vi "sv_Calculate Chirp Time and Phase Relation within Block.vi"(6 "# of even-angle samples in":i32, 10 "block size [samples]":i32, 11 "continuous swept-sine settings":T1={"amplitude"=0.0, "frequency range"={"start (Hz)"=20.0, "stop (Hz)"=20000.0, "frequency spacing"=enum."Logarithmic"}, "sampling info"={"Fs"=50000.0, "chirp duration [s]"=3.0}, "initial states"={"frequency [Hz]"=20.0, "phase [rad]"=0.0, "elapsed time [s]"=0.0}, "frequency slope"=0.0, "maximum harmonic"=0, "prefix len [samples]"={"integer"=0, "fractional"=0.0}} {"frequency slope" format="%.2f"; "prefix len [samples]"."fractional" format="%.2p"; "initial states"."elapsed time [s]" format="%.2f"; "initial states"."phase [rad]" format="%.2f"; "initial states"."frequency [Hz]" format="%.2f"; "sampling info"."chirp duration [s]" format="%.2f"; "sampling info"."Fs" format="%.2p"; "frequency range"."stop (Hz)" format="%.2f"; "frequency range"."start (Hz)" format="%.2f"; "amplitude" format="%.2f"}) -> (0 "samples/rev":i32, 1 "time instances [s]":dbl[](array[numeric]), 2 "phases [rad]":dbl[](array[numeric]), 3 "continuous swept-sine settings out":T1={"amplitude"=0.0, "frequency range"={"start (Hz)"=20.0, "stop (Hz)"=20000.0, "frequency spacing"=enum."Logarithmic"}, "sampling info"={"Fs"=50000.0, "chirp duration [s]"=3.0}, "initial states"={"frequency [Hz]"=20.0, "phase [rad]"=0.0, "elapsed time [s]"=0.0}, "frequency slope"=0.0, "maximum harmonic"=0, "prefix len [samples]"={"integer"=0, "fractional"=0.0}} {"frequency slope" format="%.2f"; "prefix len [samples]"."fractional" format="%.2p"; "initial states"."elapsed time [s]" format="%.2f"; "initial states"."phase [rad]" format="%.2f"; "initial states"."frequency [Hz]" format="%.2f"; "sampling info"."chirp duration [s]" format="%.2f"; "sampling info"."Fs" format="%.2p"; "frequency range"."stop (Hz)" format="%.2f"; "frequency range"."start (Hz)" format="%.2f"; "amplitude" format="%.2f"}, 4 "# of even-angle samples out":i32)   [LabVIEW 2017, in "SoundVib_ContSweptSine.lvlib"]
uses:
  <vilib>/addons/Sound and Vibration/svt_Continuous Swept Sine/SoundVib_ContSweptSine.lvlib
  <vilib>/addons/_NISVFA/_Generation/subVIs/sv_Chirp Settings.ctl
  <vilib>/Analysis/1siggen.llb/Ramp Pattern by Samples.vi
  <vilib>/addons/_NISVFA/_Generation/SoundVib_Generation.lvlib
  <vilib>/Analysis/NI_AALBase.lvlib
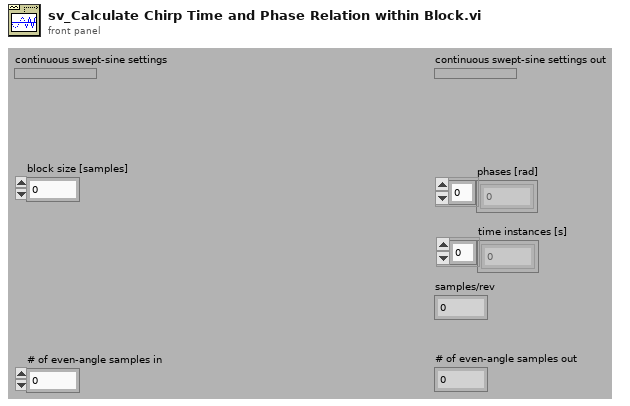
[diagram p1: front panel]
types:
  T1 = typedef "SoundVib_Generation.lvlib/sv_Chirp Settings.ctl" = cluster{"amplitude":dbl, "frequency range":cluster{"start (Hz)":dbl, "stop (Hz)":dbl, "frequency spacing":enum16{"Linear", "Logarithmic"}}, "sampling info":cluster{"Fs":dbl, "chirp duration [s]":dbl}, "initial states":cluster{"frequency [Hz]":dbl, "phase [rad]":dbl, "elapsed time [s]":dbl}, "frequency slope":dbl, "maximum harmonic":i32, "prefix len [samples]":cluster{"integer":u32, "fractional":dbl}}
  T2 = cluster{"frequency [Hz]":dbl, "phase [rad]":dbl, "elapsed time [s]":dbl}
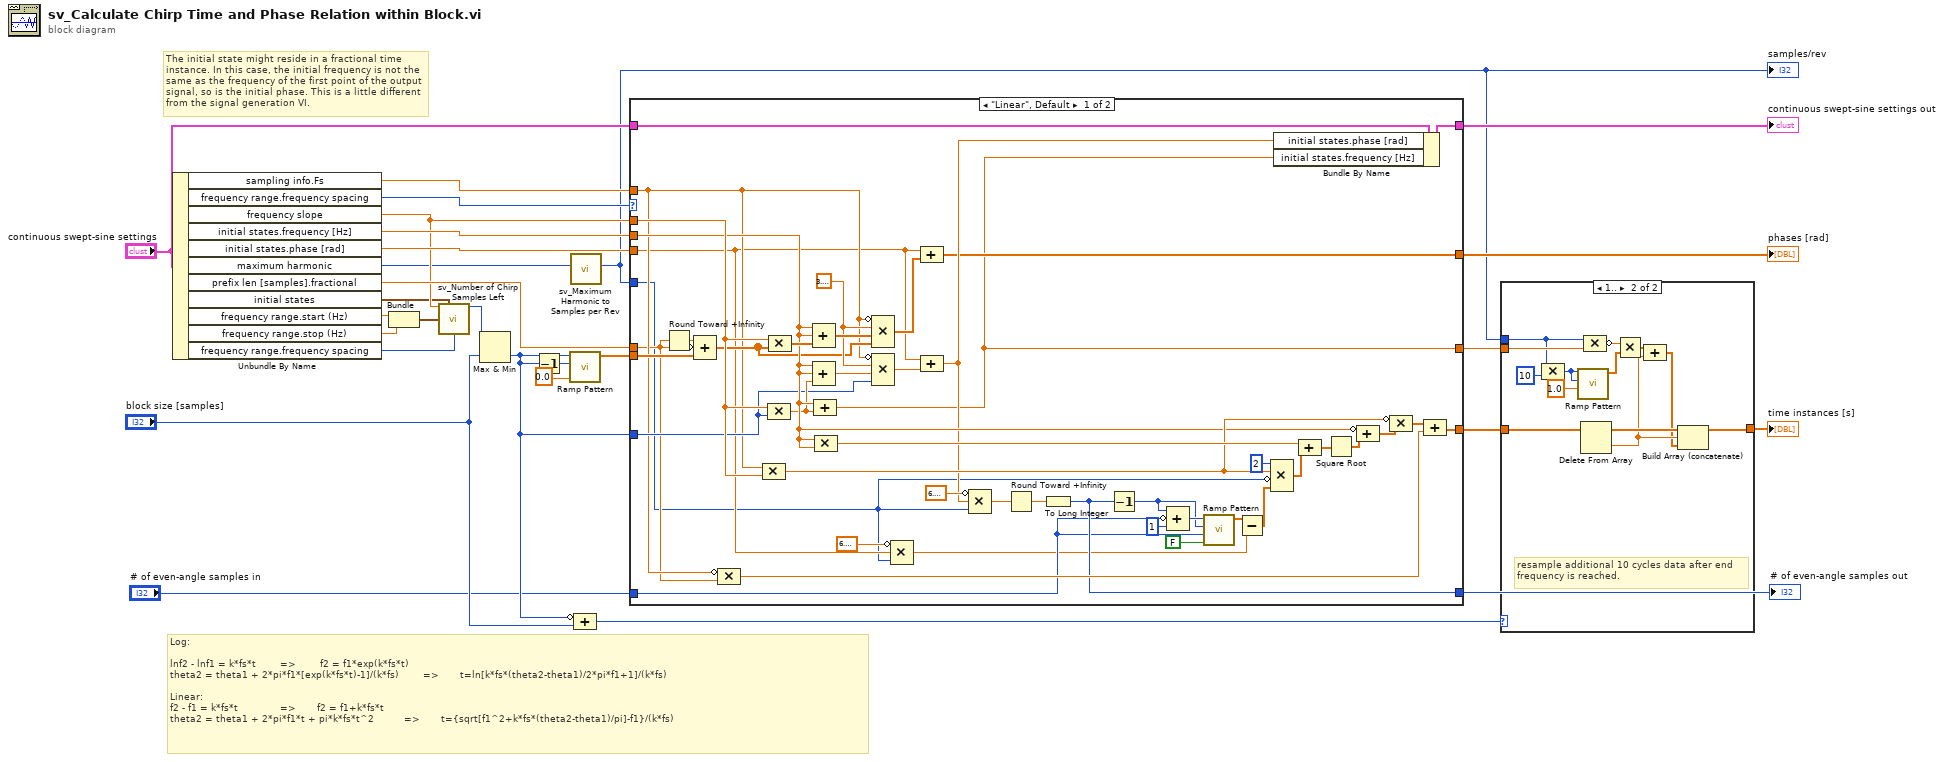
[diagram p0: block diagram]
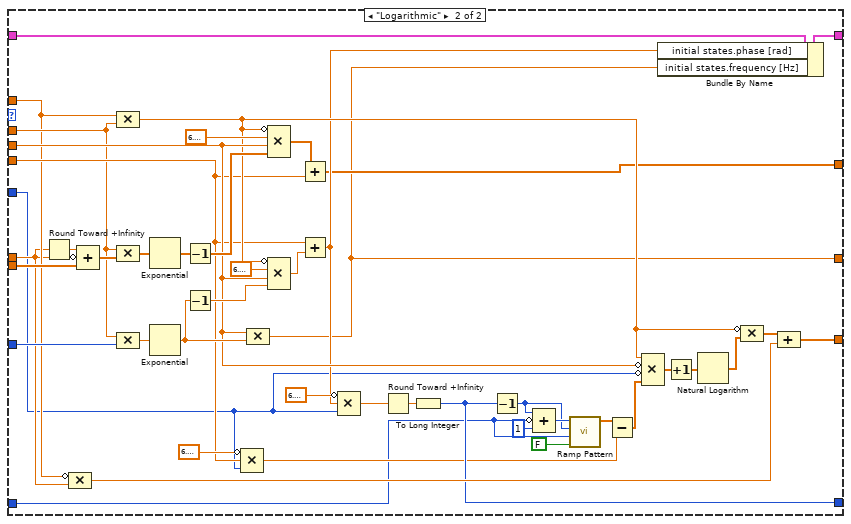
[diagram p3: hidden frame]
diagram:
  # "The initial state might reside in a fractional time instance. In this case, the initial frequency is not the same as the frequency of the first point of the output signal, so is the initial phase. This is a little different from the signal generation VI."
  # "Log:\n            \nlnf2 - lnf1 = k*fs*t        =>        f2 = f1*exp(k*fs*t)\ntheta2 = theta1 + 2*pi*f1*[exp(k*fs*t)-1]/(k*fs)        =>       t=ln[k*fs*(theta2-theta1)/2*pi*f1+1]/(k*fs)\n\nLinear:\nf2 - f1 = k*fs*t              =>       f2 = f1+k*fs*t\ntheta2 = theta1 + 2*pi*f1*t + pi*k*fs*t^2          =>       t={sqrt[f1^2+k*fs*(theta2-theta1)/pi]-f1}/(k*fs)"
  n1 = Unbundle By Name("continuous swept-sine settings") -> ("sampling info.Fs"=w16:dbl, "frequency range.frequency spacing"=w28:enum16{"Linear", "Logarithmic"}, "frequency slope"=w19:dbl, "initial states.frequency [Hz]"=w27:dbl, "initial states.phase [rad]"=w26:dbl, "maximum harmonic"=w4:i32, "prefix len [samples].fractional"=w21:dbl, "initial states"=w18:T2, "frequency range.start (Hz)"=w7:dbl, "frequency range.stop (Hz)"=w6:dbl, "frequency range.frequency spacing"=w5:enum16{"Linear", "Logarithmic"})
  n2 = Bundle("start (Hz)"=w7, "stop (Hz)"=w6) -> (w8:cluster{"start (Hz)":dbl, "stop (Hz)":dbl})  [unwired: 1 in]
  n3 = call <vilib>:"sv_Number of Chirp Samples Left.vi"("frequency slope"=w19, "initial states"=w18, "frequency range"=w8, "frequency spacing"=w5) -> ("# of samples left"=w17:i32)  [unwired: 9 in, 2 out]
  n4 = Max & Min(x=w17, y="block size [samples]") -> (min(x,y)=w14:i32)  [unwired: 1 out]
  n5 = Decrement(x=w14) -> (x-1=w20:i32)
  n6 = call-poly <vilib>:"Ramp Pattern.vi"("start"=0.0, "end"=w20, "samples"=w14) -> ("Ramp Pattern"=w24:dbl[])  [unwired: 7 in, 1 out]
  n7 = call <vilib>:"sv_Maximum Harmonic to Samples per Rev.vi"("maximum harmonic"=w4) -> ("samples/rev"=w3:i32)  [unwired: 10 in]
  "samples/rev" <- w3
  n8 = Compound Arithmetic op=ADD(invert w14, "block size [samples]") -> (w12:i32)
  n9 = case shown="\"Linear\", Default" w28 {
    tunnel: w27 -> [w53 w96]
    tunnel: w26 -> [w36 w93]
    tunnel: w19 -> [w62 w83]
    tunnel: w24 -> [w43 w115]
    tunnel: "continuous swept-sine settings" -> [w71 w116]
    tunnel: [w45 w90] -> w15
    tunnel: w14 -> [w47 w114]
    tunnel: [w70 w110] -> w22
    tunnel: w16 -> [w39 w82]
    tunnel: w3 -> [w30 w76]
    tunnel: [w42 w86] -> w10
    tunnel: w21 -> [w38 w81]
    tunnel: [w37 w80] -> w11
    tunnel: [w32 w77] -> w2
    tunnel: "# of even-angle samples in" -> [w31 w74]
    frame "Linear", Default {
      w49 = 3.141592653589793
      n10 = Round Toward +Infinity(x=w38) -> (ceil(x): smallest int >= x=w40:dbl)
      n11 = Compound Arithmetic op=ADD(w40, invert w38, w43) -> (w44:dbl[])
      n12 = Compound Arithmetic op=MULTIPLY(invert w39, w38) -> (w41:dbl)
      n13 = Compound Arithmetic op=MULTIPLY(w39, w62) -> (w55:dbl)
      n14 = Compound Arithmetic op=MULTIPLY(w62, w47) -> (w50:dbl)
      n15 = Compound Arithmetic op=MULTIPLY(w62, w44) -> (w73:dbl[])
      n16 = Compound Arithmetic op=ADD(w53, w53, w73) -> (w72:dbl[])
      n17 = Compound Arithmetic op=ADD(w53, w53, w50) -> (w51:dbl)
      n18 = Compound Arithmetic op=ADD(w53, w50) -> (w37:dbl)
      n19 = Compound Arithmetic op=MULTIPLY(w53, w53) -> (w60:dbl)
      n20 = Compound Arithmetic op=MULTIPLY(invert w39, w49, w72, w44) -> (w52:dbl[])
      n21 = Compound Arithmetic op=MULTIPLY(invert w39, w49, w51, w47) -> (w48:dbl)
      n22 = Compound Arithmetic op=MULTIPLY(invert 6.283185307179586, w36, w30) -> (w29:dbl)
      n23 = Compound Arithmetic op=ADD(w36, w52) -> (w45:dbl[])
      n24 = Compound Arithmetic op=ADD(w36, w48) -> (w46:dbl)
      n25 = Compound Arithmetic op=MULTIPLY(invert 6.283185307179586, w46, w30) -> (w35:dbl)
      n26 = Round Toward +Infinity(x=w35) -> (ceil(x): smallest int >= x=w34:dbl)
      n27 = To Long Integer(number=w34) -> (32bit integer=w32:i32)
      n28 = Decrement(x=w32) -> (x-1=w33:i32)
      n29 = Compound Arithmetic op=ADD(w33, invert w31, 1 ("value")) -> (w66:i32)
      n30 = call-poly <vilib>:"Ramp Pattern.vi"("exclude end?"=FALSE, "start"=w31, "end"=w33, "samples"=w66) -> ("Ramp Pattern"=w64:dbl[])  [unwired: 6 in, 1 out]
      n31 = Subtract(x=w64, y=w29) -> (x-y=w63:dbl[])
      n32 = Compound Arithmetic op=MULTIPLY(2, w55, invert w30, w63) -> (w59:dbl[])
      n33 = Bundle By Name(cluster=w71, "initial states.phase [rad]"=w46, "initial states.frequency [Hz]"=w37) -> (w70:T1)
      n34 = Compound Arithmetic op=ADD(w60, w59) -> (w58:dbl[])
      n35 = Square Root(x=w58) -> (sqrt(x)=w57:dbl[])
      n36 = Compound Arithmetic op=ADD(invert w53, w57) -> (w56:dbl[])
      n37 = Compound Arithmetic op=MULTIPLY(invert w55, w56) -> (w54:dbl[])
      n38 = Compound Arithmetic op=ADD(w54, w41) -> (w42:dbl[])
    }
    frame "Logarithmic" {
      n39 = Round Toward +Infinity(x=w81) -> (ceil(x): smallest int >= x=w85:dbl)
      n40 = Compound Arithmetic op=MULTIPLY(invert w82, w81) -> (w87:dbl)
      n41 = Compound Arithmetic op=ADD(w85, invert w81, w115) -> (w89:dbl[])
      n42 = Compound Arithmetic op=MULTIPLY(w82, w83) -> (w94:dbl)
      n43 = Compound Arithmetic op=MULTIPLY(w83, w89) -> (w118:dbl[])
      n44 = Compound Arithmetic op=MULTIPLY(w83, w114) -> (w112:dbl)
      n45 = Exponential(1:w118) -> (0:w113:dbl[])
      n46 = Exponential(1:w112) -> (0:w98:dbl)
      n47 = Decrement(x=w113) -> (x-1=w111:dbl[])
      n48 = Decrement(x=w98) -> (x-1=w97:dbl)
      n49 = Compound Arithmetic op=MULTIPLY(invert 6.283185307179586, w93, w76) -> (w75:dbl)
      n50 = Compound Arithmetic op=MULTIPLY(w96, w98) -> (w80:dbl)
      n51 = Compound Arithmetic op=MULTIPLY(invert w94, 6.283185307179586, w96, w111) -> (w84:dbl[])
      n52 = Compound Arithmetic op=MULTIPLY(invert w94, 6.283185307179586, w96, w97) -> (w92:dbl)
      n53 = Add(x=w84, y=w93) -> (x+y=w90:dbl[])
      n54 = Add(x=w93, y=w92) -> (x+y=w91:dbl)
      n55 = Compound Arithmetic op=MULTIPLY(invert 6.283185307179586, w91, w76) -> (w79:dbl)
      n56 = Round Toward +Infinity(x=w79) -> (ceil(x): smallest int >= x=w107:dbl)
      n57 = To Long Integer(number=w107) -> (32bit integer=w77:i32)
      n58 = Decrement(x=w77) -> (x-1=w78:i32)
      n59 = Compound Arithmetic op=ADD(w78, invert w74, 1 ("value")) -> (w105:i32)
      n60 = call-poly <vilib>:"Ramp Pattern.vi"("exclude end?"=FALSE, "start"=w74, "end"=w78, "samples"=w105) -> ("Ramp Pattern"=w103:dbl[])  [unwired: 6 in, 1 out]
      n61 = Subtract(x=w103, y=w75) -> (x-y=w99:dbl[])
      n62 = Compound Arithmetic op=MULTIPLY(w94, invert w96, invert w76, w99) -> (w102:dbl[])
      n63 = Bundle By Name(cluster=w116, "initial states.phase [rad]"=w91, "initial states.frequency [Hz]"=w80) -> (w110:T1)
      n64 = Increment(x=w102) -> (x+1=w101:dbl[])
      n65 = Natural Logarithm(1:w101) -> (0:w100:dbl[])
      n66 = Compound Arithmetic op=MULTIPLY(invert w94, w100) -> (w88:dbl[])
      n67 = Compound Arithmetic op=ADD(w88, w87) -> (w86:dbl[])
    }
  }
  "continuous swept-sine settings out" <- w22
  "phases [rad]" <- w15
  "# of even-angle samples out" <- w2
  n68 = case shown="1.." w12 {
    tunnel: w11 -> [_ w132]
    tunnel: w3 -> [_ w130]
    tunnel: w10 -> [w119 w125]
    tunnel: [w119 w120] -> w9
    frame 0, Default {
    }
    frame 1.. {
      # "resample additional 10 cycles data after end\nfrequency is reached."
      n69 = Compound Arithmetic op=MULTIPLY(w130, 10 ("samples")) -> (w129:i32)
      n70 = call-poly <vilib>:"Ramp Pattern.vi"("start"=1.0, "end"=w129, "samples"=w129) -> ("Ramp Pattern"=w126:dbl[])  [unwired: 7 in, 1 out]
      n71 = Delete From Array(array=w125) -> (deleted portion=w122:dbl, array with subset deleted=w123:dbl[])  [unwired: 2 in]
      n72 = Compound Arithmetic op=MULTIPLY(w130, w132) -> (invert w127:dbl)
      n73 = Multiply(x=w127, y=w126) -> (x*y=w124:dbl[])
      n74 = Compound Arithmetic op=ADD(w124, w122) -> (w121:dbl[])
      n75 = Build Array (concatenate)(w123, w122, w121) -> (w120:dbl[])
    }
  }
  "time instances [s]" <- w9
